vi "GoTo_a.vi"(11 "VISA resource name":refnum<visa-resource-name>="COM7") -> (2 "read string":string)   [LabVIEW 2017]
uses:
  controls/#typedef_Queue Cmd.ctl
panel:
  in  "Position":u8
  in  "Go To Button":bool
  in  "Callib Button":bool
  out "error out":errorcluster
  in  "error in (no error)":errorcluster
  in  "stop":bool
  in  "Get ID Button":bool
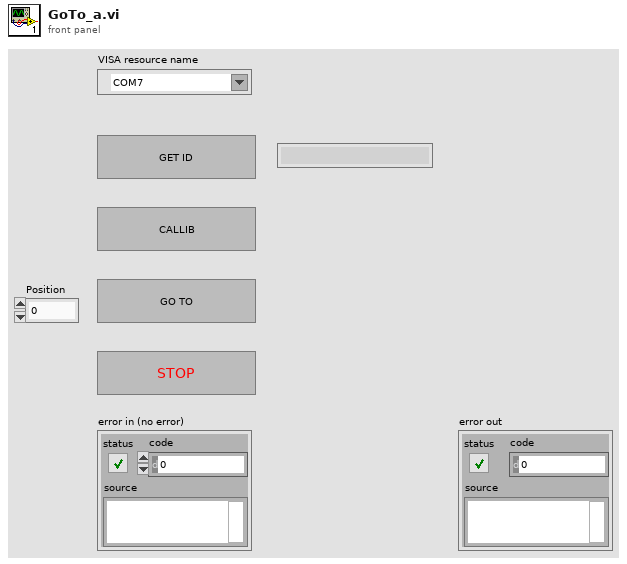
[diagram p1: front panel]
types:
  T1 = typedef "#typedef_Queue Cmd.ctl" = enum16{"Get ID", "Callib", "Go to", "Exit"}
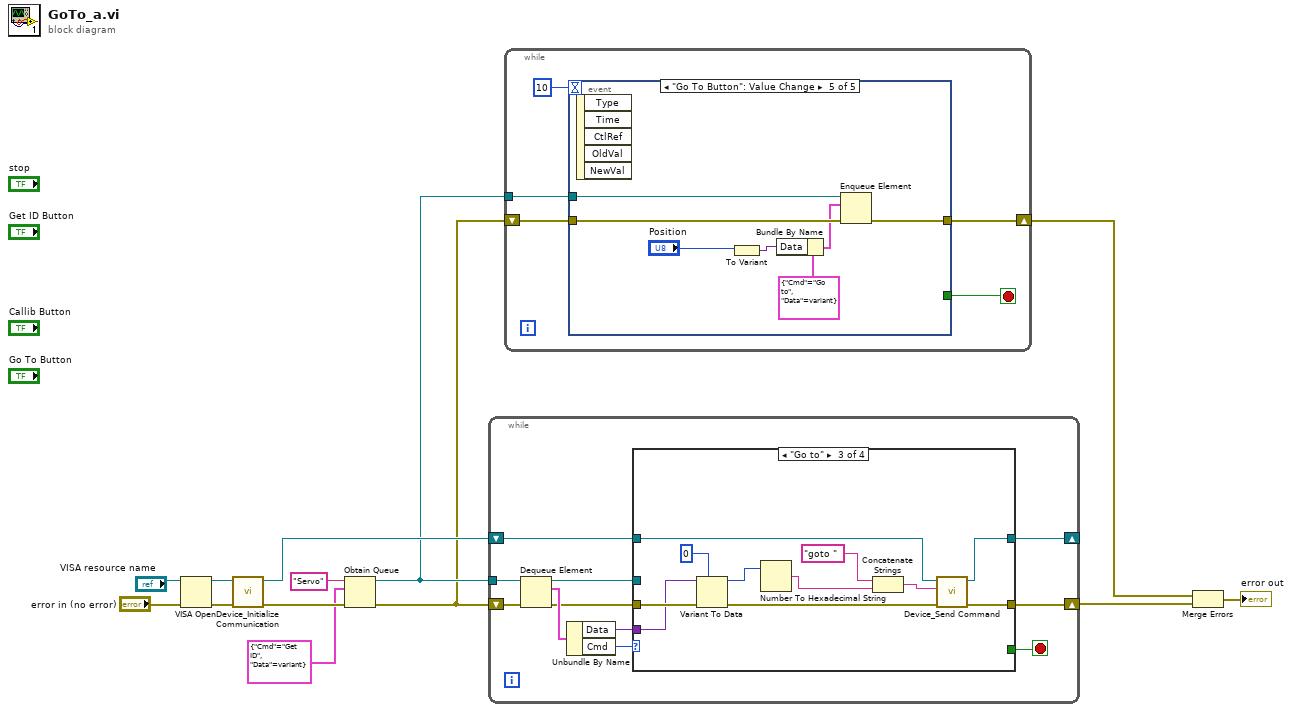
[diagram p0: block diagram]
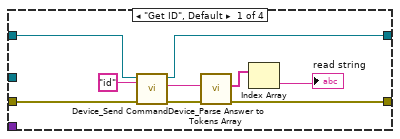
[diagram p2: hidden frame]
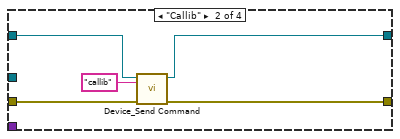
[diagram p3: hidden frame]
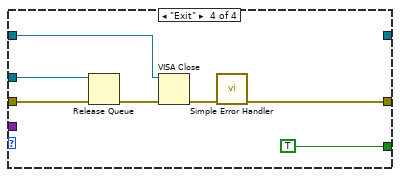
[diagram p4: hidden frame]
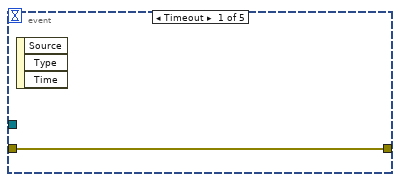
[diagram p5: hidden frame]
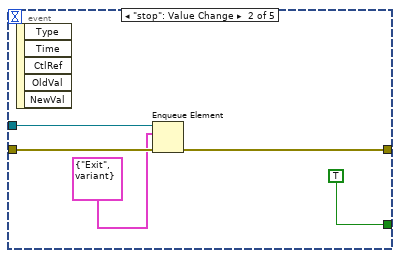
[diagram p6: hidden frame]
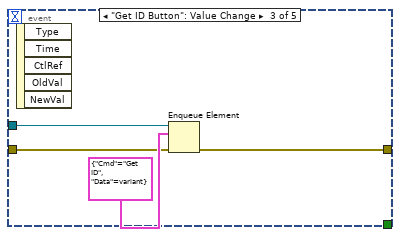
[diagram p7: hidden frame]
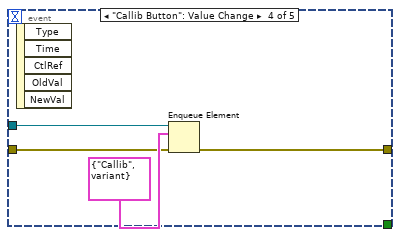
[diagram p8: hidden frame]
diagram:
  n1 = VISA Open(error in (no error)="error in (no error)", VISA resource name="VISA resource name") -> (VISA resource name=w12:refnum<visa-resource-name>, error out=w11:errorcluster)  [unwired: 3 in]
  n2 = call "Device_Initialize Communication.vi"("error in (no error)"=w11, "VISA Refnum in"=w12) -> ("error out"=w9:errorcluster, "VISA Refnum out"=w8:refnum<visa-resource-name>)  [unwired: 8 in]
  n3 = Obtain Queue(name (unnamed)="Servo", element data type=cluster{"Cmd":T1, "Data":variant} {"Cmd"=enum."Get ID", "Data"=variant} ("Queue Msg"), error in (no error)=w9) -> (queue out=w5:refnum<queue>, error out=w4:errorcluster)  [unwired: 2 in, 1 out]
  n4 = while {
    shift-right: [w15] -> _
    shift-left: w8 -> [w16]
    tunnel: w5 -> [w23]
    shift-right: [w18] -> w3
    shift-left: w4 -> [w24]
    stop <- w17 stop-if-true
    n5 = Dequeue Element(queue=w23, error in (no error)=w24) -> (queue out=w19:refnum<queue>, element=w22:cluster{"Cmd":T1, "Data":variant}, error out=w20:errorcluster)  [unwired: 1 in, 1 out]
    n6 = Unbundle By Name(w22) -> ("Data"=w14:variant, "Cmd"=w21:T1)
    n7 = case shown="\"Go to\"" w21 {
      tunnel: w20 -> [w31 w36 w46 w56]
      tunnel: w19 -> [_ _ _ w55]
      tunnel: [w28 w34 w47 w50] -> w18
      tunnel: [_ _ _ TRUE] -> w17
      tunnel: w16 -> [w32 w37 w49 w52]
      tunnel: [w30 w35 w48 _] -> w15
      tunnel: w14 -> [_ _ w43 _]
      frame "Get ID", Default {
        n8 = call "Device_Send Command.vi"("error in (no error)"=w31, "write string"="id", "VISA Refnum in"=w32) -> ("error out"=w29:errorcluster, "read buffer"=w27:string, "VISA Refnum out"=w30:refnum<visa-resource-name>)  [unwired: 6 in]
        n9 = call "Device_Parse Answer to Tokens Array.vi"("error in (no error)"=w29, "Answer"=w27) -> ("error out"=w28:errorcluster, "Tokens Array"=w26:string[])  [unwired: 8 in]
        n10 = Index Array(array=w26) -> (element=→"read string":string)  [unwired: 1 in]
      }
      frame "Callib" {
        n11 = call "Device_Send Command.vi"("error in (no error)"=w36, "write string"="callib", "VISA Refnum in"=w37) -> ("error out"=w34:errorcluster, "VISA Refnum out"=w35:refnum<visa-resource-name>)  [unwired: 6 in, 1 out]
      }
      frame "Go to" {
        n12 = Variant To Data(error in=w46, type=u8 0 ("Position 2"), Variant=w43) -> (data=w42:u8, error out=w45:errorcluster)
        n13 = Number To Hexadecimal String(2:w42) -> (0:w40:string)  [unwired: 1 in]
        n14 = Concatenate Strings("goto " ("write string"), w40) -> (w39:string)
        n15 = call "Device_Send Command.vi"("error in (no error)"=w45, "write string"=w39, "VISA Refnum in"=w49) -> ("error out"=w47:errorcluster, "VISA Refnum out"=w48:refnum<visa-resource-name>)  [unwired: 6 in, 1 out]
      }
      frame "Exit" {
        n16 = Release Queue(queue=w55, error in (no error)=w56) -> (error out=w51:errorcluster)  [unwired: 1 in, 2 out]
        n17 = VISA Close(VISA resource name=w52, error in (no error)=w51) -> (error out=w53:errorcluster)
        n18 = call <vilib>:"Simple Error Handler.vi"("error in (no error)"=w53) -> ("error out"=w50:errorcluster)  [unwired: 4 in, 4 out]
      }
    }
  }
  n19 = while {
    tunnel: w5 -> [w61]
    shift-right: [w59] -> w2
    shift-left: w4 -> [w60]
    stop <- w58 stop-if-true
    n20 = event shown="[4] \"Go To Button\": Value Change" {
      selector: _ -> [_ _ _ _ _]
      dyn-events: _ -> [_ _ _ _ _]
      timeout: 10 -> [_ _ _ _ _]
      tunnel: w61 -> [_ w64 w69 w73 w81]
      tunnel: w60 -> [w62 w67 w70 w74 w82]
      tunnel: [w62 w66 w68 w72 w80] -> w59
      tunnel: [_ TRUE _ _ _] -> w58
      event Timeout {
        n21 = event-data() -> ()  [unwired: 1 in, 3 out]
      }
      event "stop": Value Change {
        n22 = event-data() -> ()  [unwired: 1 in, 5 out]
        n23 = Enqueue Element(queue=w64, element=cluster{"Cmd":T1, "Data":variant} {"Cmd"=enum."Exit", "Data"=variant} ("Queue Msg"), error in (no error)=w67) -> (error out=w66:errorcluster)  [unwired: 1 in, 2 out]
      }
      event "Get ID Button": Value Change {
        n24 = event-data() -> ()  [unwired: 1 in, 5 out]
        n25 = Enqueue Element(queue=w69, element=cluster{"Cmd":T1, "Data":variant} {"Cmd"=enum."Get ID", "Data"=variant} ("Queue Msg"), error in (no error)=w70) -> (error out=w68:errorcluster)  [unwired: 1 in, 2 out]
      }
      event "Callib Button": Value Change {
        n26 = event-data() -> ()  [unwired: 1 in, 5 out]
        n27 = Enqueue Element(queue=w73, element=cluster{"Cmd":T1, "Data":variant} {"Cmd"=enum."Callib", "Data"=variant} ("Queue Msg"), error in (no error)=w74) -> (error out=w72:errorcluster)  [unwired: 1 in, 2 out]
      }
      event "Go To Button": Value Change {
        n28 = event-data() -> ()  [unwired: 1 in, 5 out]
        n29 = To Variant(anything="Position") -> (Variant=w77:variant)
        n30 = Bundle By Name(cluster=cluster{"Cmd":T1, "Data":variant} {"Cmd"=enum."Go to", "Data"=variant} ("Queue Msg"), "Data"=w77) -> (w78:cluster{"Cmd":T1, "Data":variant})
        n31 = Enqueue Element(queue=w81, element=w78, error in (no error)=w82) -> (error out=w80:errorcluster)  [unwired: 1 in, 2 out]
      }
    }
  }
  n32 = Merge Errors(w2, w3) -> (→"error out":errorcluster)
